vi "ReadAndSaveData.vi"(0 "object in":refnum<class "InstrumentBase.lvclass">, 1 "tdms file":refnum<k34>, 2 "group name in (Untitled)":string, 5 "error in (no error)":errorcluster) -> (14 "object out":refnum<class "InstrumentBase.lvclass">, 15 "Channels array":waveform(dbl)[](array[waveform]), 16 "output cluster":T1, 19 "error out":errorcluster)   [LabVIEW 2023, in "InstrumentBase.lvclass"]
uses:
  InstrumentBase.lvclass
  InstrumentBase.lvclass/InstrumentBase.ctl
  <vilib>/measure/NI_MAPro.lvlib
  <vilib>/measure/matone.llb/Extract Single Tone Information 1 Chan.vi
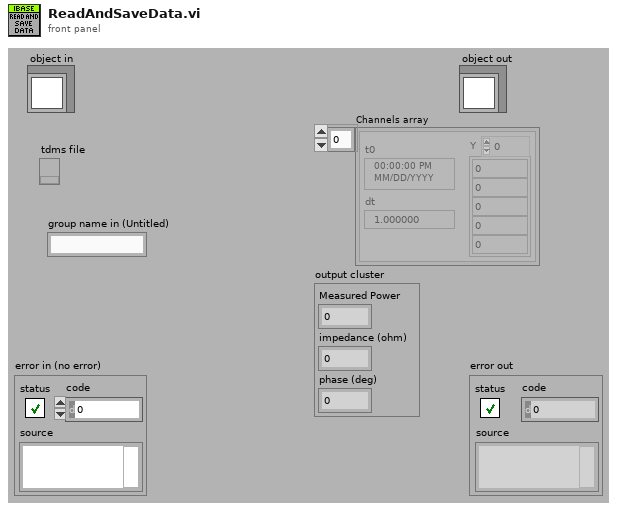
[diagram p1: front panel]
types:
  T1 = cluster{"Measured Power":dbl, "impedance (ohm)":dbl, "phase (deg)":dbl}
  T2 = cluster{"Config.Ch1.Carrier.Frequency (Hz)":dbl, "Config.Ch2.Carrier.Frequency (Hz)":dbl, "Config.Ch1.Carrier.Amplitude (V)":dbl, "Config.Ch2.Carrier.Amplitude (V)":dbl}
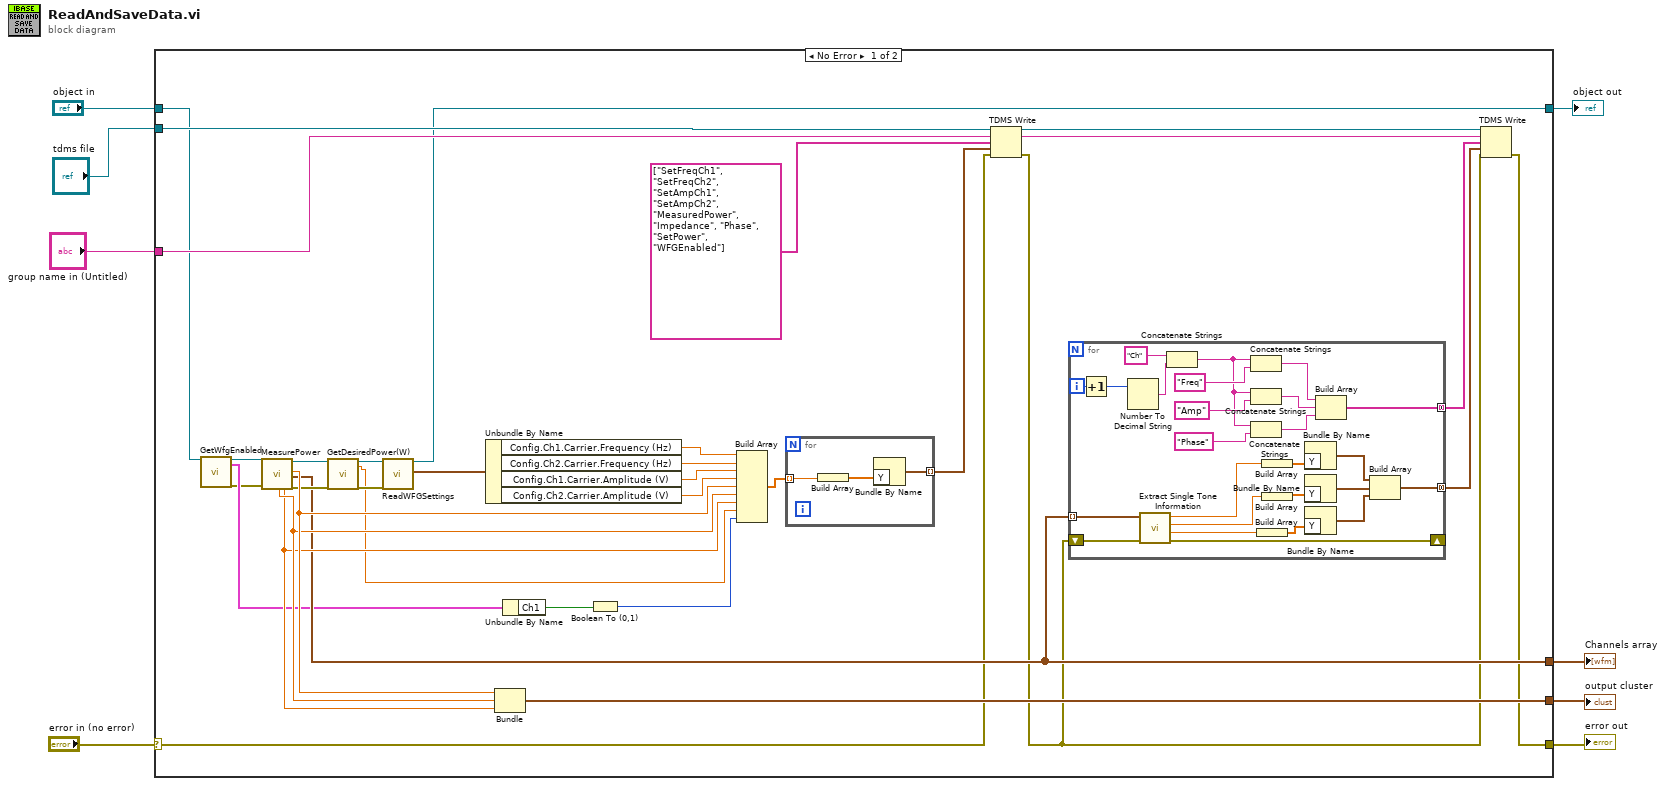
[diagram p0: block diagram]
diagram:
  n1 = case shown="No Error" "error in (no error)" {
    selector: "error in (no error)" -> [w20 w72]
    tunnel: [w18 w72] -> w7
    tunnel: [w10 w71] -> w5
    tunnel: "object in" -> [w9 w71]
    tunnel: "tdms file" -> [w42 _]
    tunnel: "group name in (Untitled)" -> [w35 _]
    tunnel: [w23 _] -> w2
    tunnel: [w32 _] -> w1
    frame No Error {
      n2 = call-dynamic "GetWfgEnabled.vi"("object in"=w9) -> ("object out"=w15:refnum<class "InstrumentBase.lvclass">, "WfgEnabled"=w14:cluster{"Ch1":bool, "Ch2":bool}, "error out"=w11:errorcluster)  [unwired: 16 in]
      n3 = call-dynamic "MeasurePower.vi"("object in"=w15, "error in (no error)"=w11) -> ("impedance (ohm)"=w30:dbl, "phase (deg)"=w29:dbl, "object out"=w27:refnum<class "InstrumentBase.lvclass">, "Measured Power"=w31:dbl, "Channels array"=w23:waveform(dbl)[], "error out"=w28:errorcluster)  [unwired: 12 in]
      n4 = call-dynamic "GetDesiredPower(W).vi"("object in"=w27, "error in (no error)"=w28) -> ("object out"=w26:refnum<class "InstrumentBase.lvclass">, "DesiredPower(W)"=w24:dbl, "error out"=w25:errorcluster)  [unwired: 15 in]
      n5 = call-dynamic "ReadWFGSettings.vi"("object in"=w26, "error in (no error)"=w25) -> ("object out"=w10:refnum<class "InstrumentBase.lvclass">, "AmplitudeAndVoltage"=w36:T2)  [unwired: 15 in, 1 out]
      n6 = Unbundle By Name(w36) -> ("Config.Ch1.Carrier.Frequency (Hz)"=w41:dbl, "Config.Ch2.Carrier.Frequency (Hz)"=w40:dbl, "Config.Ch1.Carrier.Amplitude (V)"=w39:dbl, "Config.Ch2.Carrier.Amplitude (V)"=w38:dbl)
      n7 = Bundle("Measured Power"=w31, "impedance (ohm)"=w30, "phase (deg)"=w29) -> (w32:T1)  [unwired: 1 in]
      n8 = Unbundle By Name(w14) -> ("Ch1"=w13:bool)
      n9 = Boolean To (0,1)(Boolean=w13) -> (0, 1=w12:i16)
      n10 = Build Array(w41, w40, w39, w38, w31, w30, w29, w24, w12) -> (w37:dbl[])
      n11 = for {
        tunnel: w37 -> [w70] mode=indexing
        tunnel: [w68] -> w33 mode=indexing
        n12 = Build Array(w70) -> (w69:dbl[])
        n13 = Bundle By Name("Y"=w69) -> (w68:waveform(dbl))  [unwired: 1 in]
      }
      n14 = TDMS Write(0:w42, 5:w35, 7:string[] ["SetFreqCh1", "SetFreqCh2", "SetAmpCh1", "SetAmpCh2", "MeasuredPower", "Impedance", "Phase", "SetPower", "WFGEnabled"] ("channel name(s) in (Untitled)"), 9:w33, 11:w20) -> (4:w17:refnum<k34>, 6:w16:string, 15:w19:errorcluster)  [unwired: 1 in, 1 out]
      n15 = for {
        tunnel: [w59] -> w22 mode=concatenating
        shift-right: [w54] -> _
        shift-left: w19 -> [w55]
        tunnel: w23 -> [w53] mode=indexing
        tunnel: [w43] -> w21 mode=concatenating
        i -> [w65]
        n16 = Increment(x=w65) -> (x+1=w60:i32)
        n17 = Number To Decimal String(number=w60) -> (decimal integer string=w66:string)  [unwired: 1 in]
        n18 = call-poly <vilib>:"Extract Single Tone Information.vi"("error in (no error)"=w55, "time signal in"=w53) -> ("error out"=w54:errorcluster, "detected phase (deg)"=w48:dbl, "detected amplitude"=w49:dbl, "detected frequency"=w52:dbl)  [unwired: 4 in, 2 out]
        n19 = Concatenate Strings("Ch" ("string"), w66) -> (w58:string)
        n20 = Concatenate Strings(w58, "Freq") -> (w62:string)
        n21 = Concatenate Strings(w58, "Amp") -> (w61:string)
        n22 = Concatenate Strings(w58, "Phase") -> (w56:string)
        n23 = Build Array(w48) -> (w50:dbl[])
        n24 = Build Array(w52) -> (w51:dbl[])
        n25 = Build Array(w49) -> (w47:dbl[])
        n26 = Bundle By Name("Y"=w51) -> (w46:waveform(dbl))  [unwired: 1 in]
        n27 = Bundle By Name("Y"=w47) -> (w45:waveform(dbl))  [unwired: 1 in]
        n28 = Bundle By Name("Y"=w50) -> (w44:waveform(dbl))  [unwired: 1 in]
        n29 = Build Array(w62, w61, w56) -> (w59:string[])
        n30 = Build Array(w46, w45, w44) -> (w43:waveform(dbl)[])
      }
      n31 = TDMS Write(0:w17, 5:w16, 7:w22, 9:w21, 11:w19) -> (15:w18:errorcluster)  [unwired: 1 in, 3 out]
    }
    frame Error {
    }
  }
  "error out" <- w7
  "object out" <- w5
  "Channels array" <- w2
  "output cluster" <- w1
